vi "NiMyDAQ.vi"() -> ()   [LabVIEW 2021]
uses:
  Main states enum-MyDAQ.ctl
  <vilib>/DAQmx/write.llb/DAQmx Write (Analog DBL 1Chan 1Samp).vi
  <vilib>/DAQmx/create/channels.llb/DAQmx Create Channel (AO-Voltage-Basic).vi
  Globals/Global message.vi
  Globals/CH1.vi
  Globals/CH2.vi
  Globals/CH3.vi
  Globals/CH4.vi
  Globals/CH5.vi
  <vilib>/DAQmx/miscellaneous.llb/DAQmx Fill In Error Info.vi
panel:
  in  "START":bool
  out "Measurand":dbl
  in  "physical channels":tag
  in  "Measurement channel":enum16{"CH1", "CH2", "CH3", "CH4", "CH5"}(ring)
  in  "Channel type":T1(ring)
  in  "Stop Button":bool
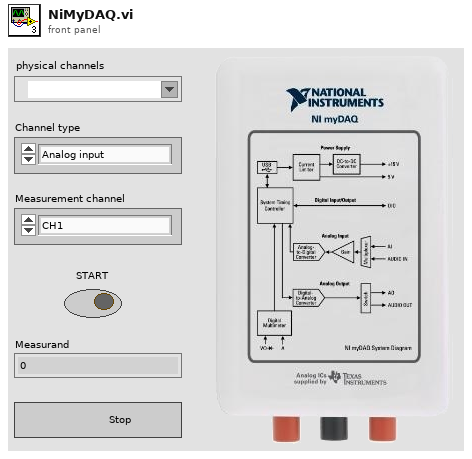
[diagram p1: front panel]
types:
  T1 = enum16{"Analog input", "Analog output", "Digital input", "Digital output", "Multimeter"}
  T2 = typedef "Main states enum-MyDAQ.ctl" = enum16{"Initialize", "Update", "Stop"}
  T3 = cluster{"Voltage":dbl, "Current":dbl, "Message":string}
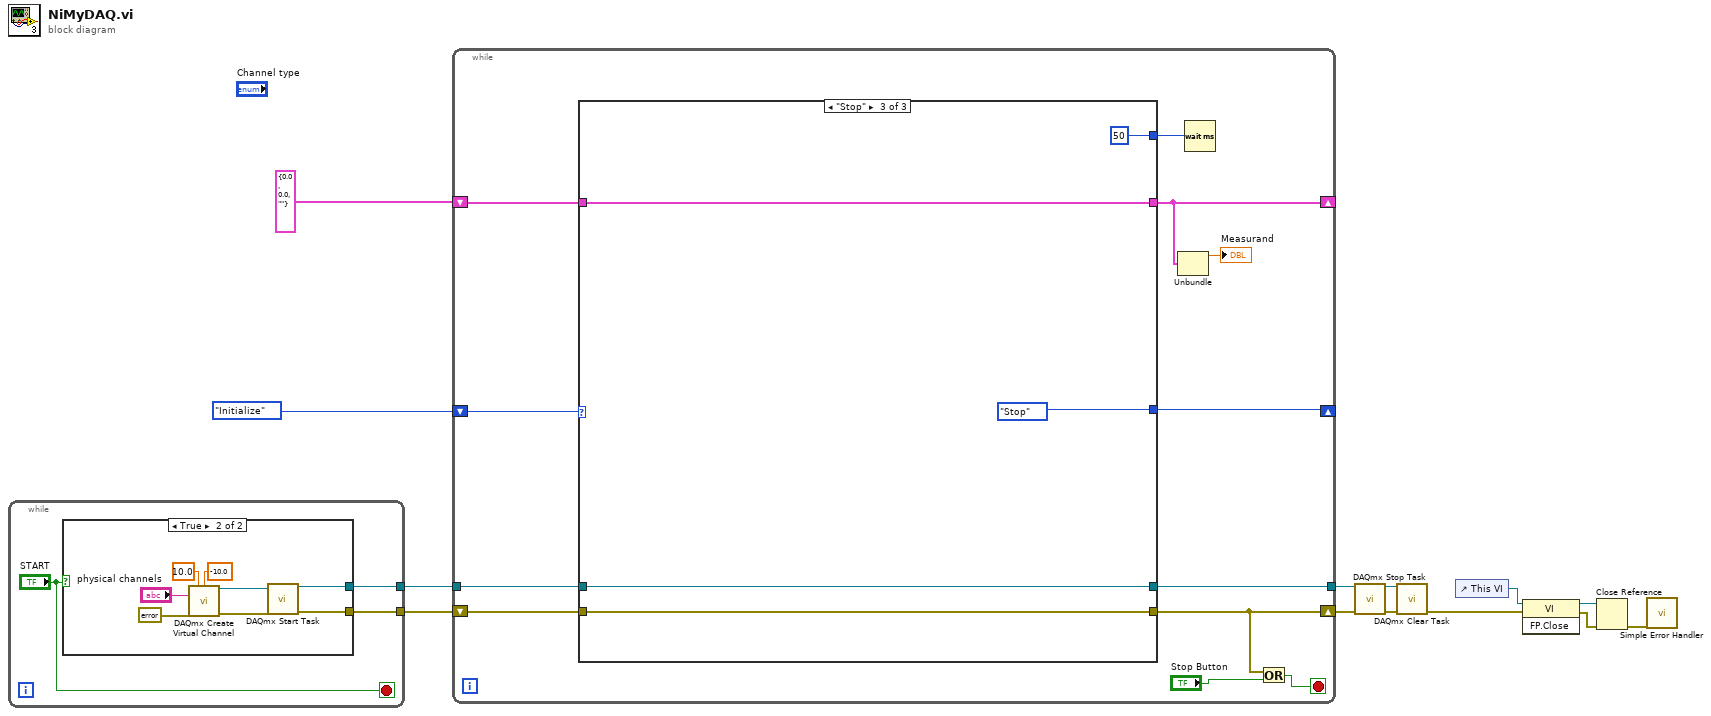
[diagram p0: block diagram]
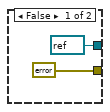
[diagram p2: hidden frame]
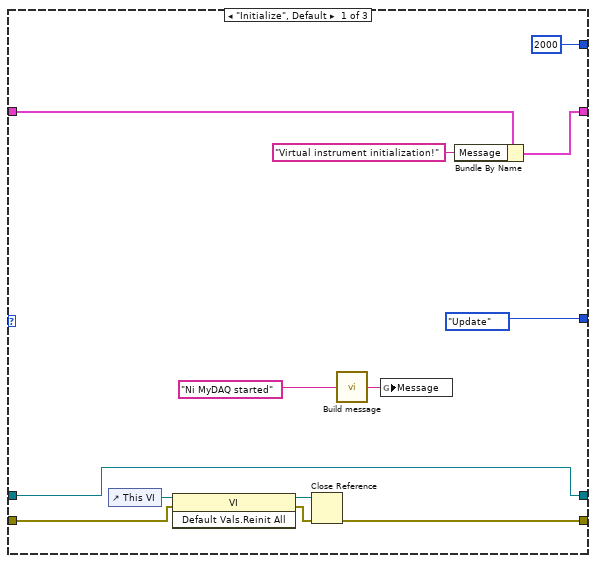
[diagram p3: hidden frame]
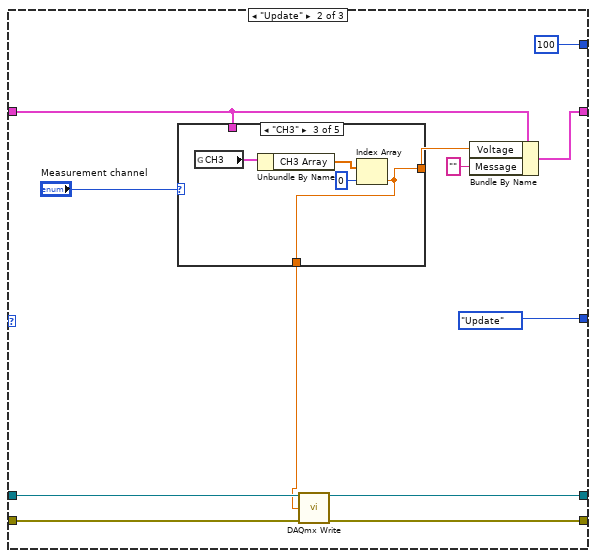
[diagram p4: hidden frame]
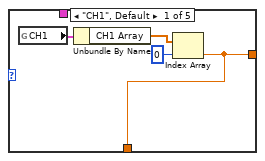
[diagram p5: hidden frame]
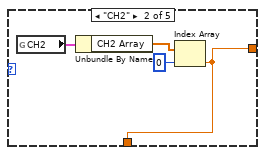
[diagram p6: hidden frame]
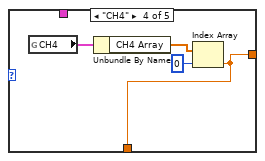
[diagram p7: hidden frame]
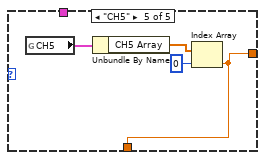
[diagram p8: hidden frame]
diagram:
  n1 = while {
    tunnel: [w16] -> w7
    tunnel: [w15] -> w6
    stop <- "START" stop-if-true
    n2 = case shown="True" "START" {
      tunnel: [errorcluster {"status"=FALSE, "code"=0, "source"=""} ("error out") w20] -> w16
      tunnel: [refnum<k21> refnum ("task out") w19] -> w15
      frame False {
      }
      frame True {
        n3 = call-poly <vilib>:"DAQmx Create Virtual Channel.vi"("maximum value"=10.0, "minimum value"=-10.0, "physical channels"="physical channels", "error in"=errorcluster {"status"=FALSE, "code"=0, "source"=""} ("error constant")) -> ("task out"=w22:refnum<k21>, "error out"=w21:errorcluster)  [unwired: 10 in]
        n4 = call <vilib>:"DAQmx Start Task.vi"("task/channels in"=w22, "error in"=w21) -> ("task out"=w19:refnum<k21>, "error out"=w20:errorcluster)  [unwired: 12 in]
      }
    }
  }
  n5 = while {
    shift-right: [w36] -> w5
    shift-left: w7 -> [w38]
    shift-right: [w32] -> _
    shift-left: T3 {"Voltage"=0.0, "Current"=0.0, "Message"=""} -> [w35]
    shift-right: [w33] -> _
    shift-left: Main_states_enum-MyDAQ."Initialize" ("Enum") -> [w34]
    tunnel: w6 -> [w29]
    tunnel: [w28] -> w4
    stop <- w37 stop-if-true
    n6 = case shown="\"Stop\"" w34 {
      tunnel: w38 -> [w48 w57 w88]
      tunnel: [w43 w56 w88] -> w36
      tunnel: w35 -> [w45 w59 w86]
      tunnel: [w44 w63 w86] -> w32
      tunnel: [Main_states_enum-MyDAQ."Update" ("Enum") Main_states_enum-MyDAQ."Update" ("Enum") Main_states_enum-MyDAQ."Stop" ("Enum")] -> w33
      tunnel: [u32 2000 ("milliseconds to wait") u32 100 ("milliseconds to wait") u32 50 ("milliseconds to wait")] -> w31
      tunnel: w29 -> [w39 w55 w84]
      tunnel: [w39 w54 w84] -> w28
      frame "Initialize", Default {
        n7 = control-ref of="This VI"() -> (w51:refnum<vi>)
        n8 = invoke class="VI" method="Default Vals.Reinit All"(reference=w51, error in=w48) -> (reference out=w50:refnum<vi>, error out=w49:errorcluster)  [unwired: 1 in, 1 out]
        n9 = Close Reference(reference=w50, error in (no error)=w49) -> (error out=w43:errorcluster)
        n10 = call "Build message.vi"("Input string"="Ni MyDAQ started") -> ("Output string"=w40:string)
        n11 = global write "Global message.vi" "Message"(w40) -> ()
        n12 = Bundle By Name(cluster=w45, "Message"="Virtual instrument initialization!") -> (w44:T3)
      }
      frame "Update" {
        n13 = case shown="\"CH3\"" "Measurement channel" {
          tunnel: [w64 w68 w72 w76 w81] -> w60
          tunnel: w59 -> [_ _ _ _ _]
          tunnel: [w64 w68 w72 w76 w81] -> w52
          frame "CH1", Default {
            n14 = global read "CH1.vi" "CH1"() -> (w67:cluster{"CH1 Array":dbl[], "CH1 Message":string})
            n15 = Unbundle By Name(w67) -> ("CH1 Array"=w66:dbl[])
            n16 = Index Array(array=w66, index=0) -> (element=w64:dbl)
          }
          frame "CH2" {
            n17 = global read "CH2.vi" "CH2"() -> (w69:cluster{"CH2 Array":dbl[], "CH2 Message":string})
            n18 = Unbundle By Name(w69) -> ("CH2 Array"=w71:dbl[])
            n19 = Index Array(array=w71, index=0) -> (element=w68:dbl)
          }
          frame "CH3" {
            n20 = global read "CH3.vi" "CH3"() -> (w73:cluster{"CH3 Array":dbl[], "CH3 Message":string})
            n21 = Unbundle By Name(w73) -> ("CH3 Array"=w75:dbl[])
            n22 = Index Array(array=w75, index=0) -> (element=w72:dbl)
          }
          frame "CH4" {
            n23 = global read "CH4.vi" "CH4"() -> (w77:cluster{"CH4 Array":dbl[], "CH4 Message":string})
            n24 = Unbundle By Name(w77) -> ("CH4 Array"=w79:dbl[])
            n25 = Index Array(array=w79, index=0) -> (element=w76:dbl)
          }
          frame "CH5" {
            n26 = global read "CH5.vi" "CH5"() -> (w80:cluster{"CH5 Array":dbl[], "CH5 Message":string})
            n27 = Unbundle By Name(w80) -> ("CH5 Array"=w83:dbl[])
            n28 = Index Array(array=w83, index=0) -> (element=w81:dbl)
          }
        }
        n29 = call-poly <vilib>:"DAQmx Write.vi"("task/channels in"=w55, "data"=w52, "error in"=w57) -> ("task out"=w54:refnum<k21>, "error out"=w56:errorcluster)  [unwired: 10 in, 1 out]
        n30 = Bundle By Name(cluster=w59, "Voltage"=w60, "Message"="") -> (w63:T3)
      }
      frame "Stop" {
      }
    }
    n31 = Unbundle(w32) -> ("Voltage"=→"Measurand":dbl)  [unwired: 2 out]
    n32 = Wait (ms)(milliseconds to wait=w31) -> ()  [unwired: 1 out]
    n33 = Or(x=w36, y="Stop Button") -> (x .or. y?=w37:bool)
  }
  n34 = call <vilib>:"DAQmx Stop Task.vi"("task/channels in"=w4, "error in"=w5) -> ("task out"=w3:refnum<k21>, "error out"=w2:errorcluster)  [unwired: 12 in]
  n35 = call <vilib>:"DAQmx Clear Task.vi"("task in"=w3, "error in"=w2) -> ("error out"=w1:errorcluster)  [unwired: 13 in]
  n36 = control-ref of="This VI"() -> (w11:refnum<vi>)
  n37 = invoke class="VI" method="FP.Close"(reference=w11, error in=w1) -> (reference out=w9:refnum<vi>, error out=w10:errorcluster)  [unwired: 1 in, 1 out]
  n38 = Close Reference(reference=w9, error in (no error)=w10) -> (error out=w13:errorcluster)
  n39 = call <vilib>:"Simple Error Handler.vi"("error in (no error)"=w13) -> ()  [unwired: 4 in, 5 out]
